vi "NI VeriStand FPGA Interface Tools Installer.vi"() -> ()   [LabVIEW 2010]
panel:
  out "Install Status":string
  in  "Uninstall":bool
  in  "Accept":bool
  out "License":string="Copyright (c) 2011, National Instruments\nAll rights reserved.\n\nRedistribution and use in source and binary forms, with or without modification, are permitted provided that the following conditions are met:\n\no Redistributions of source code must retain the above copyright notice, this list of conditions and the following disclaimer.\no Redistributions in binary form must reproduce the above copyright notice, this list of conditions and the following disclaimer in the documentation and/or other materials provided with the distribution.\no Neither the name of the National Instruments Corporation nor the names of its contributors may be used to endorse or promote products derived from this software without specific prior written permission.\n\nTHIS SOFTWARE IS PROVIDED BY THE COPYRIGHT HOLDERS AND CONTRIBUTORS \"AS IS\" AND ANY EXPRESS OR IMPLIED WARRANTIES, INCLUDING, BUT NOT LIMITED TO, THE IMPLIED WARRANTIES OF MERCHANTABILITY AND FITNESS FOR A PARTICULAR PURPOSE ARE DISCLAIMED. IN NO EVENT SHALL THE COPYRIGHT HOLDER OR CONTRIBUTORS BE LIABLE FOR ANY DIRECT, INDIRECT, INCIDENTAL, SPECIAL, EXEMPLARY, OR CONSEQUENTIAL DAMAGES (INCLUDING, BUT NOT LIMITED TO, PROCUREMENT OF SUBSTITUTE GOODS OR SERVICES; LOSS OF USE, DATA, OR PROFITS; OR BUSINESS INTERRUPTION) HOWEVER CAUSED AND ON ANY THEORY OF LIABILITY, WHETHER IN CONTRACT, STRICT LIABILITY, OR TORT (INCLUDING NEGLIGENCE OR OTHERWISE) ARISING IN ANY WAY OUT OF THE USE OF THIS SOFTWARE, EVEN IF ADVISED OF THE POSSIBILITY OF SUCH DAMAGE."
  in  "Cancel":bool
  in  "Install":bool
  # "NI VeriStand FPGA-Based I/O Interface Tools"
  # "1. Installs NI VeriStand FPGA project wizard to Getting Started Windows and New dialog.\n2. Installs NI VeriStand RIO Library, NI VeriStand FPGA Templates, palettes, and examples."
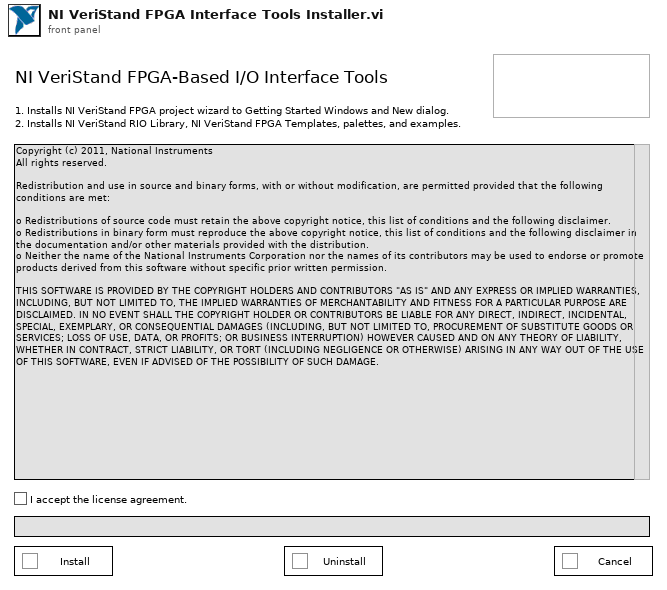
[diagram p1: front panel]
types:
  T1 = enum8{"Enabled", "Disabled", "Disabled and Grayed Out"}
  T2 = enum16{"copy files", "Xplatform copy", "move external linked files to temp", "mass compile", "move temp files to user.lib", "del mass comp proj"}
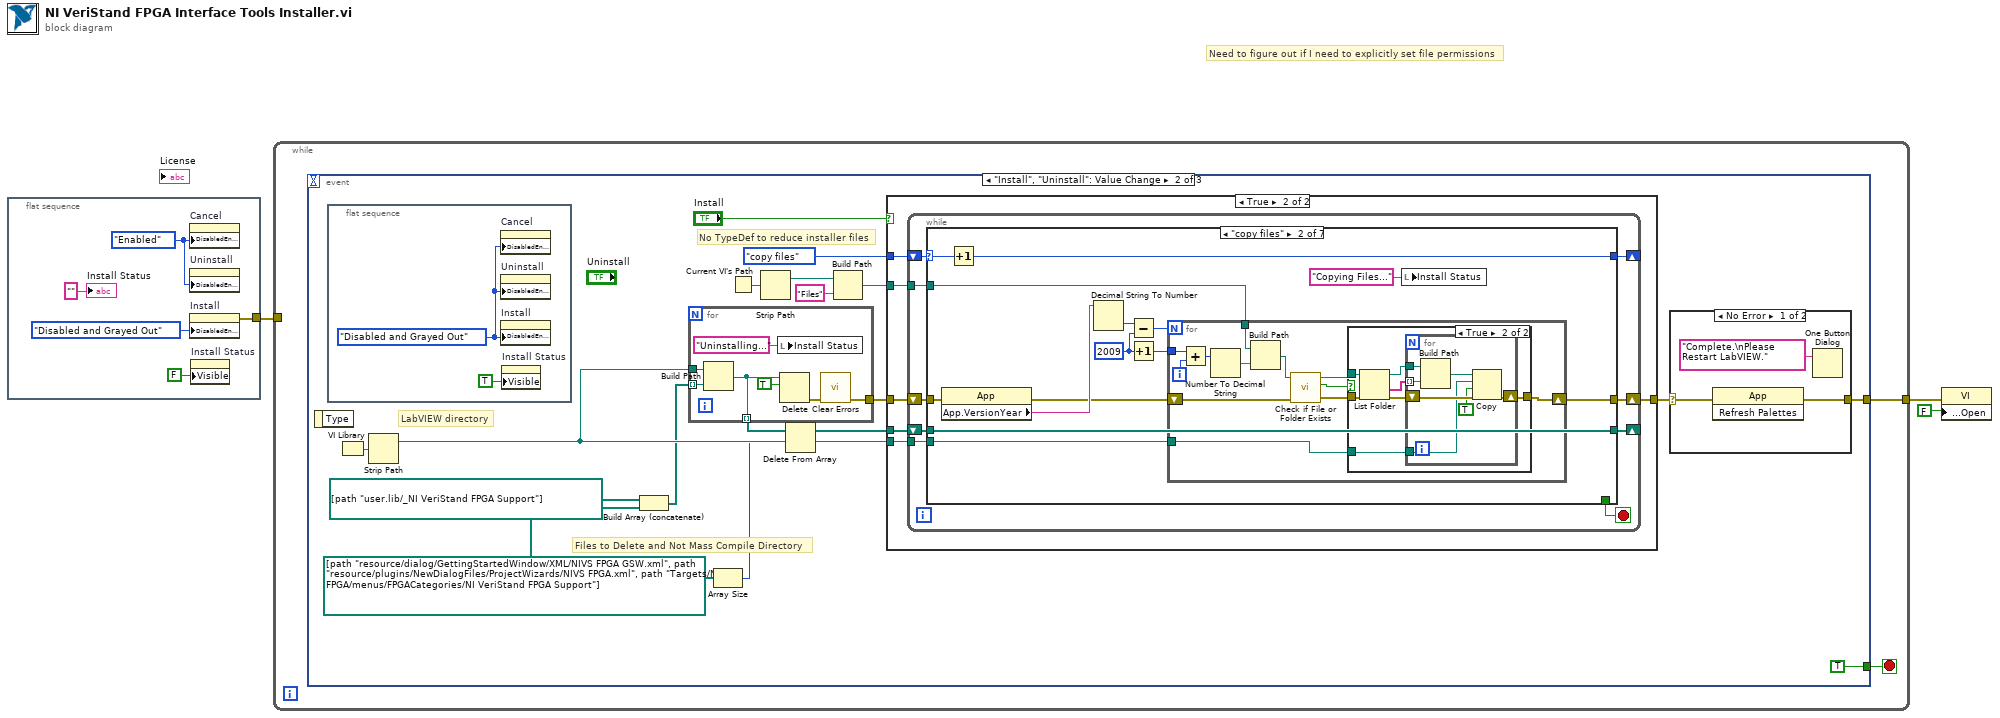
[diagram p0: block diagram]
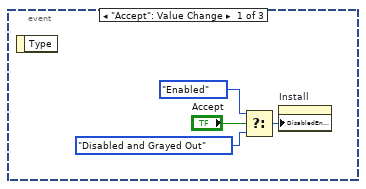
[diagram p2: hidden frame]
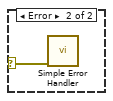
[diagram p3: hidden frame]
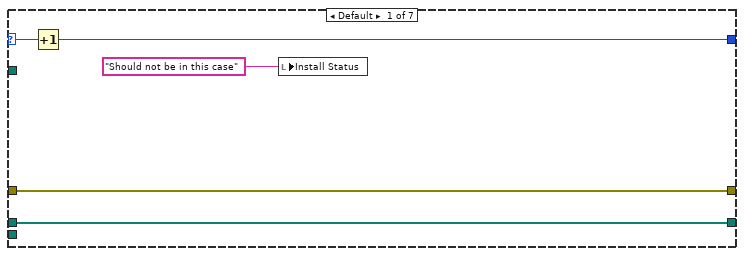
[diagram p5: hidden frame]
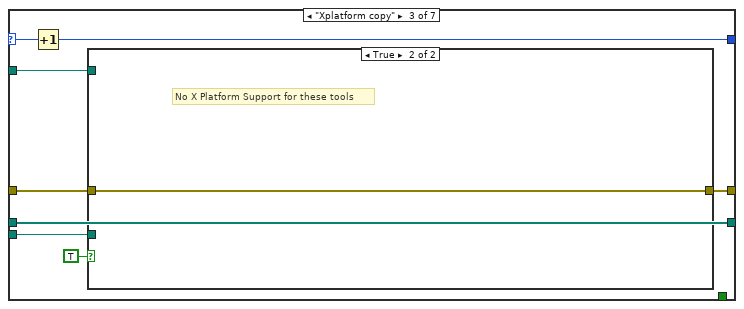
[diagram p7: hidden frame]
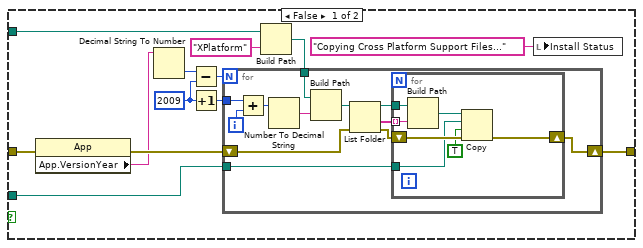
[diagram p8: hidden frame]
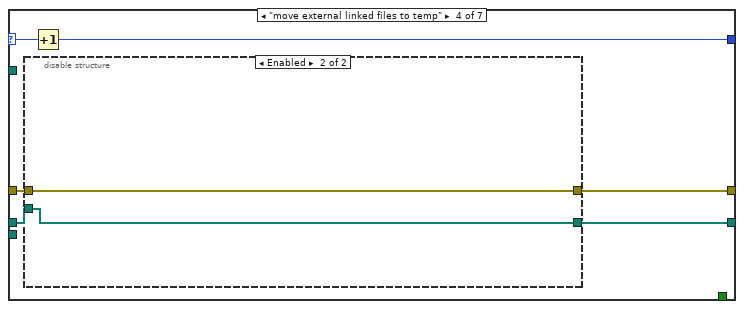
[diagram p9: hidden frame]
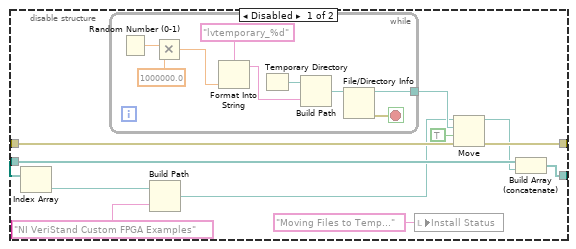
[diagram p10: hidden frame]
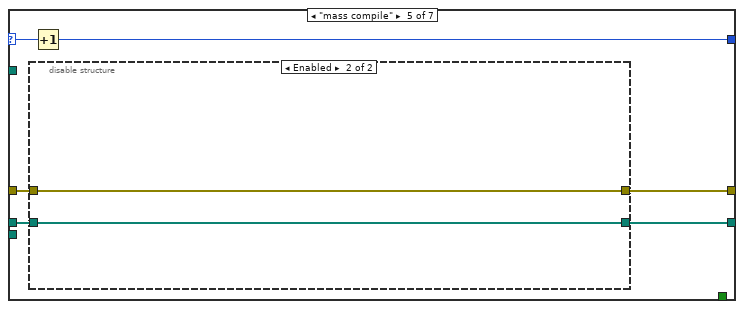
[diagram p11: hidden frame]
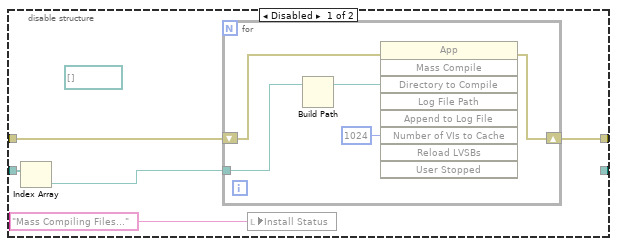
[diagram p12: hidden frame]
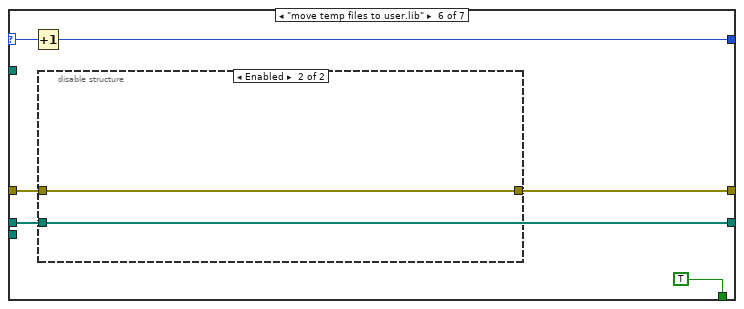
[diagram p13: hidden frame]
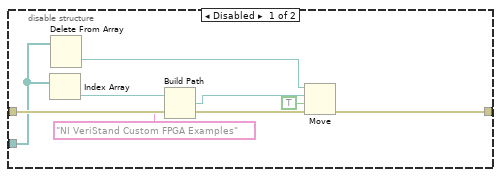
[diagram p14: hidden frame]
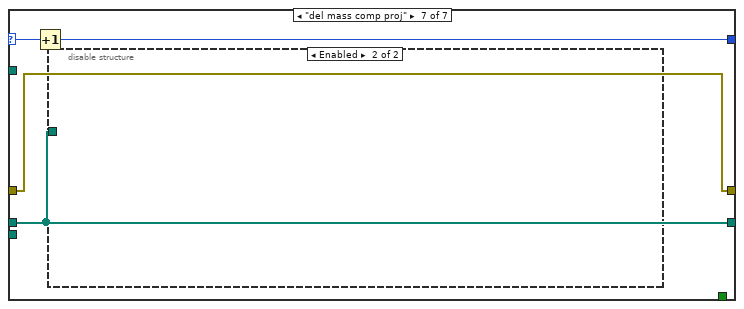
[diagram p15: hidden frame]
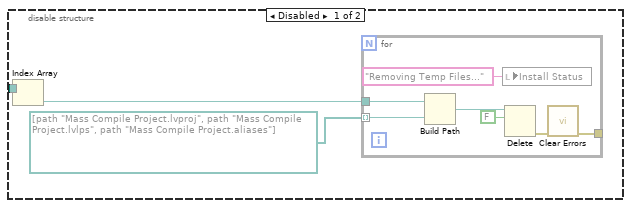
[diagram p16: hidden frame]
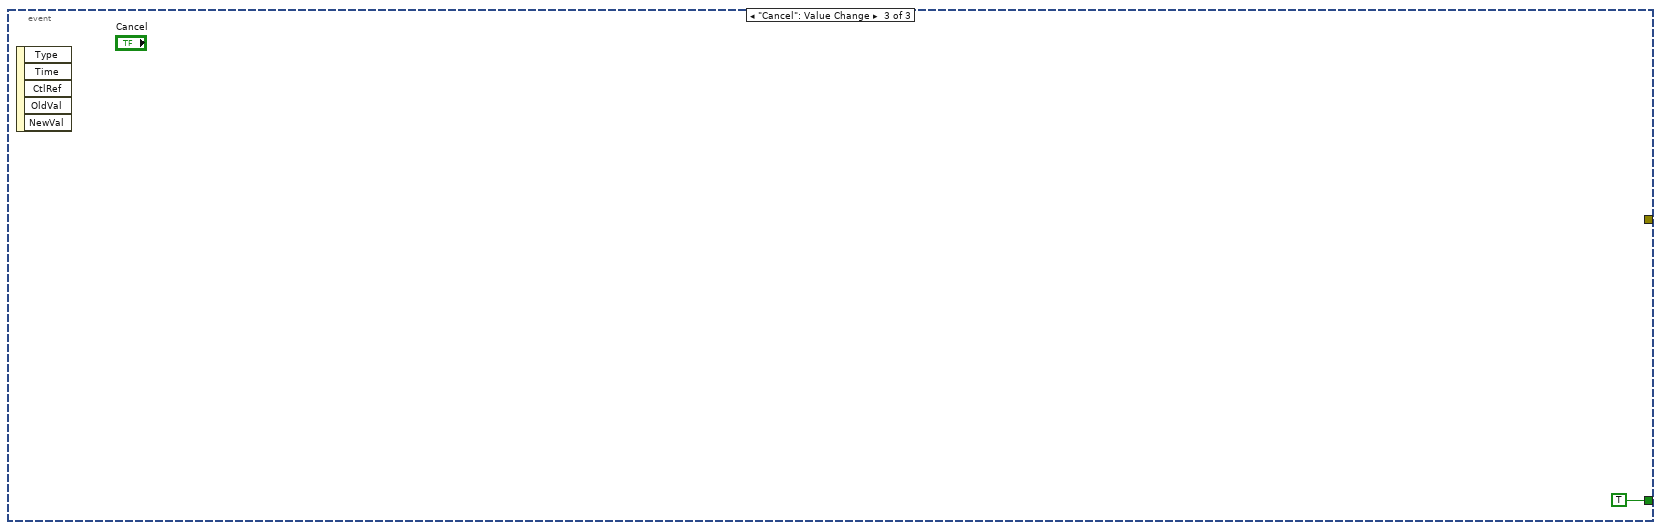
[diagram p17: hidden frame]
diagram:
  # "Need to figure out if I need to explicitly set file permissions"
  n1 = flat-sequence {
    tunnel: [w4] -> w3
    frame #0 {
      w8 = T1."Enabled" ("Disabled")
      n2 = property on="Cancel" class="Bool"("DisabledEnum"=w8) -> ()  [unwired: 2 in, 2 out]
      n3 = property on="Uninstall" class="Bool"("DisabledEnum"=w8) -> ()  [unwired: 2 in, 2 out]
      n4 = property on="Install" class="Bool"("DisabledEnum"=T1."Disabled and Grayed Out" ("Disabled")) -> (error out=w4:errorcluster)  [unwired: 2 in, 1 out]
      n5 = property on="Install Status" class="Str"("Visible"=FALSE) -> ()  [unwired: 2 in, 2 out]
      "Install Status" <- "" ("Install Status")
    }
  }
  n6 = while {
    tunnel: w3 -> [_]
    tunnel: [w9] -> w1
    stop <- w10 stop-if-true
    n7 = event shown="[1] \"Install\", \"Uninstall\": Value Change" {
      selector: _ -> [_ _ _]
      dyn-events: _ -> [_ _ _]
      timeout: _ -> [_ _ _]
      tunnel: [_ TRUE TRUE] -> w10
      tunnel: [_ w21 _] -> w9
      event "Accept": Value Change {
        n8 = event-data() -> ()  [unwired: 1 in, 1 out]
        n9 = Select(t=T1."Enabled" ("Disabled"), s="Accept", f=T1."Disabled and Grayed Out" ("Disabled")) -> (s? t:f=w12:T1)
        n10 = property on="Install" class="Bool"("DisabledEnum"=w12) -> ()  [unwired: 2 in, 2 out]
      }
      event "Install", "Uninstall": Value Change {
        w17 = path[] [path "resource/dialog/GettingStartedWindow/XML/NIVS FPGA GSW.xml", path "resource/plugins/NewDialogFiles/ProjectWizards/NIVS FPGA.xml", path "Targets/NI/FPGA/menus/FPGACategories/NI VeriStand FPGA Support"] ("element")
        # "Files to Delete and Not Mass Compile Directory"
        # "No TypeDef to reduce installer files"
        # "LabVIEW directory"
        n11 = event-data() -> ()  [unwired: 1 in, 1 out]
        n12 = flat-sequence {
          frame #0 {
            w223 = T1."Disabled and Grayed Out" ("Disabled")
            n13 = property on="Cancel" class="Bool"("DisabledEnum"=w223) -> ()  [unwired: 2 in, 2 out]
            n14 = property on="Uninstall" class="Bool"("DisabledEnum"=w223) -> ()  [unwired: 2 in, 2 out]
            n15 = property on="Install" class="Bool"("DisabledEnum"=w223) -> ()  [unwired: 2 in, 2 out]
            n16 = property on="Install Status" class="Str"("Visible"=TRUE) -> ()  [unwired: 2 in, 2 out]
          }
        }
        n17 = VI Library() -> (path=w31:path)
        n18 = Strip Path(path=w31) -> (stripped path=w23:path)  [unwired: 1 out]
        n19 = Build Array (concatenate)(path[] [path "user.lib/_NI VeriStand FPGA Support"], w17) -> (w19:path[])
        n20 = for {
          tunnel: w23 -> [w221]
          tunnel: w19 -> [w220] mode=indexing
          tunnel: [w216] -> w24
          tunnel: [w215] -> w20 mode=indexing
          n21 = Build Path(base path=w221, name or relative path=w220) -> (appended path=w215:path)
          n22 = local write "Install Status"("Uninstalling..." ("Install Status")) -> ()
          n23 = Delete(path (use dialog)=w215, entire hierarchy (F)=TRUE) -> (error out=w217:errorcluster)  [unwired: 3 in, 2 out]
          n24 = call <vilib>:"Clear Errors.vi"("error in (no error)"=w217) -> ("error out"=w216:errorcluster)  [unwired: 6 in]
        }
        n25 = Array Size(array=w17) -> (size(s)=w16:i32)
        n26 = Current VI's Path() -> (path=w30:path)
        n27 = Strip Path(path=w30) -> (stripped path=w29:path)  [unwired: 1 out]
        n28 = Delete From Array(array=w20, length=w16) -> (array with subset deleted=w18:path[])  [unwired: 1 in, 1 out]
        n29 = Build Path(base path=w29, name or relative path="Files") -> (appended path=w25:path)
        n30 = case shown="True" "Install" {
          tunnel: T2."copy files" -> [_ w43]
          tunnel: w25 -> [_ w42]
          tunnel: w24 -> [w37 w41]
          tunnel: w23 -> [_ w40]
          tunnel: w18 -> [_ w39]
          tunnel: [w37 w38] -> w22
          frame False {
          }
          frame True {
            n31 = while {
              shift-right: [w51] -> _
              shift-left: w43 -> [w52]
              tunnel: w42 -> [w49]
              shift-right: [w46] -> w38
              shift-left: w41 -> [w48]
              tunnel: w40 -> [w47]
              shift-right: [w44] -> _
              shift-left: w39 -> [w45]
              stop <- w50 stop-if-true
              n32 = case shown="\"copy files\"" w52 {
                selector: w52 -> [w57 w71 w106 w145 w173 w191 w204]
                tunnel: [w56 w70 w105 w144 w172 w190 w203] -> w51
                tunnel: [_ _ _ _ _ TRUE _] -> w50
                tunnel: w49 -> [_ w63 w104 _ _ _ _]
                tunnel: w48 -> [w53 w69 w101 w142 w171 w188 w201]
                tunnel: w47 -> [_ w62 w103 _ _ _ _]
                tunnel: [w53 w60 w102 w141 w170 w187 w201] -> w46
                tunnel: w45 -> [w54 w58 w100 w143 w169 w186 w202]
                tunnel: [w54 w58 w100 w140 w168 w186 w202] -> w44
                frame Default {
                  n33 = Increment(x=w57) -> (x+1=w56:T2)
                  n34 = local write "Install Status"("Should not be in this case" ("Install Status")) -> ()
                }
                frame "copy files" {
                  w65 = 2009 ("y")
                  n35 = property class="App"(error in=w69) -> (error out=w61:errorcluster, "App.VersionYear"=w68:string)  [unwired: 1 in, 1 out]
                  n36 = Increment(x=w71) -> (x+1=w70:T2)
                  n37 = Decimal String To Number(string=w68) -> (number=w67:i32)  [unwired: 2 in, 1 out]
                  n38 = Subtract(x=w67, y=w65) -> (x-y=w66:i32)
                  n39 = Increment(x=w65) -> (x+1=w64:i32)
                  n40 = for {
                    N: w66 -> [_]
                    tunnel: w64 -> [w83]
                    tunnel: w63 -> [w79]
                    tunnel: w62 -> [w78]
                    shift-right: [w76] -> w60
                    shift-left: w61 -> [w77]
                    i -> [w82]
                    n41 = Add(x=w83, y=w82) -> (x+y=w81:i32)
                    n42 = Number To Decimal String(number=w81) -> (decimal integer string=w80:string)  [unwired: 1 in]
                    n43 = Build Path(base path=w79, name or relative path=w80) -> (appended path=w74:path)
                    n44 = call <vilib>:"Check if File or Folder Exists.vi"("error in (no error)"=w77, "path"=w74) -> ("error out"=w75:errorcluster, "file or folder exists?"=w72:bool, "dup path"=w73:path)  [unwired: 7 in]
                    n45 = case shown="True" w72 {
                      tunnel: w73 -> [_ w88]
                      tunnel: w78 -> [_ w87]
                      tunnel: w75 -> [w84 w86]
                      tunnel: [w84 w85] -> w76
                      frame False {
                      }
                      frame True {
                        n46 = List Folder(path=w88, error in=w86) -> (path out=w90:path, folder names=w89:string[], error out=w91:errorcluster)  [unwired: 2 in, 1 out]
                        n47 = for {
                          tunnel: w89 -> [w97] mode=indexing
                          tunnel: w90 -> [w98]
                          shift-right: [w92] -> w85
                          shift-left: w91 -> [w95]
                          tunnel: w87 -> [w93]
                          n48 = Build Path(base path=w98, name or relative path=w97) -> (appended path=w96:path)
                          n49 = Copy(8:w95, 9:TRUE ("overwrite (F)"), 10:w93, 11:w96) -> (0:w92:errorcluster)  [unwired: 1 in, 2 out]
                        }
                      }
                    }
                  }
                  n50 = local write "Install Status"("Copying Files..." ("Install Status")) -> ()
                }
                frame "Xplatform copy" {
                  n51 = Increment(x=w106) -> (x+1=w105:T2)
                  n52 = case shown="True" TRUE {
                    tunnel: w104 -> [w112 _]
                    tunnel: w103 -> [w115 _]
                    tunnel: w101 -> [w109 w139]
                    tunnel: [w114 w139] -> w102
                    frame False {
                      w117 = 2009 ("y")
                      n53 = property class="App"(error in=w109) -> (error out=w108:errorcluster, "App.VersionYear"=w107:string)  [unwired: 1 in, 1 out]
                      n54 = Decimal String To Number(string=w107) -> (number=w119:i32)  [unwired: 2 in, 1 out]
                      n55 = Subtract(x=w119, y=w117) -> (x-y=w118:i32)
                      n56 = Increment(x=w117) -> (x+1=w116:i32)
                      n57 = Build Path(base path=w112, name or relative path="XPlatform") -> (appended path=w111:path)
                      n58 = for {
                        N: w118 -> [_]
                        tunnel: w116 -> [w131]
                        tunnel: w111 -> [w127]
                        tunnel: w115 -> [w122]
                        shift-right: [w120] -> w114
                        shift-left: w108 -> [w121]
                        i -> [w130]
                        n59 = Add(x=w131, y=w130) -> (x+y=w129:i32)
                        n60 = Number To Decimal String(number=w129) -> (decimal integer string=w128:string)  [unwired: 1 in]
                        n61 = Build Path(base path=w127, name or relative path=w128) -> (appended path=w123:path)
                        n62 = List Folder(path=w123, error in=w121) -> (path out=w125:path, folder names=w124:string[], error out=w126:errorcluster)  [unwired: 2 in, 1 out]
                        n63 = for {
                          tunnel: w124 -> [w137] mode=indexing
                          tunnel: w125 -> [w138]
                          shift-right: [w132] -> w120
                          shift-left: w126 -> [w135]
                          tunnel: w122 -> [w133]
                          n64 = Build Path(base path=w138, name or relative path=w137) -> (appended path=w136:path)
                          n65 = Copy(8:w135, 9:TRUE ("overwrite (F)"), 10:w133, 11:w136) -> (0:w132:errorcluster)  [unwired: 1 in, 2 out]
                        }
                      }
                      n66 = local write "Install Status"("Copying Cross Platform Support Files..." ("Install Status")) -> ()
                    }
                    frame True {
                      # "No X Platform Support for these tools"
                    }
                  }
                }
                frame "move external linked files to temp" {
                  n67 = disable-structure shown="Enabled" {
                    disable-tunnel: w143 -> [w156 w167]
                    disable-tunnel: w142 -> [w155 w166]
                    disable-tunnel: [w154 w166] -> w141
                    disable-tunnel: [w153 w167] -> w140
                    frame Disabled {
                      n68 = Index Array(array=w156) -> (element=w152:path)  [unwired: 1 in]
                      n69 = while {
                        tunnel: [w157] -> w150
                        stop <- w158 stop-if-true
                        n70 = Random Number (0-1)() -> (number: 0 to 1=w165:dbl)
                        n71 = Multiply(x=w165, y=1000000.0) -> (x*y=w162:dbl)
                        n72 = Format Into String(format string="lvtemporary_%d", w162) -> (resulting string=w161:string)  [unwired: 2 in, 1 out]
                        n73 = Temporary Directory() -> (w160:path)
                        n74 = Build Path(base path=w160, name or relative path=w161) -> (appended path=w159:path)
                        n75 = File/Directory Info(path=w159) -> (path out=w157:path, error out=w158:errorcluster)  [unwired: 1 in, 5 out]
                      }
                      n76 = Build Path(base path=w152, name or relative path="NI VeriStand Custom FPGA Examples") -> (appended path=w149:path)
                      n77 = local write "Install Status"("Moving Files to Temp..." ("Install Status")) -> ()
                      n78 = Move(source path=w149, error in=w155, 9:TRUE ("overwrite (F)"), 10:w150) -> (error out=w154:errorcluster, 3:w147:path)  [unwired: 1 in, 1 out]
                      n79 = Build Array (concatenate)(w156, w147) -> (w153:path[])
                    }
                    frame Enabled {
                    }
                  }
                  n80 = Increment(x=w145) -> (x+1=w144:T2)
                }
                frame "mass compile" {
                  n81 = disable-structure shown="Enabled" {
                    disable-tunnel: w171 -> [w177 w184]
                    disable-tunnel: [w176 w184] -> w170
                    disable-tunnel: w169 -> [w175 w185]
                    disable-tunnel: [_ w185] -> w168
                    frame Disabled {
                      (unwired) path[] []
                      n82 = Index Array(array=w175) -> (element=w174:path)  [unwired: 1 in]
                      n83 = for {
                        shift-right: [w182] -> w176
                        shift-left: w177 -> [w183]
                        tunnel: w174 -> [w179]
                        n84 = Build Path(base path=w179) -> (appended path=w180:path)  [unwired: 1 in]
                        n85 = invoke class="App" method="Mass Compile"(error in=w183, "Directory to Compile"=w180, "Number of VIs to Cache"=u32 1024) -> (error out=w182:errorcluster)  [unwired: 6 in, 8 out]
                      }
                      n86 = local write "Install Status"("Mass Compiling Files..." ("Install Status")) -> ()
                    }
                    frame Enabled {
                    }
                  }
                  n87 = Increment(x=w173) -> (x+1=w172:T2)
                }
                frame "move temp files to user.lib" {
                  n88 = Increment(x=w191) -> (x+1=w190:T2)
                  n89 = disable-structure shown="Enabled" {
                    disable-tunnel: w188 -> [w199 w200]
                    disable-tunnel: [w198 w200] -> w187
                    disable-tunnel: w186 -> [w197 _]
                    frame Disabled {
                      n90 = Index Array(array=w197) -> (element=w194:path)  [unwired: 1 in]
                      n91 = Delete From Array(array=w197) -> (deleted portion=w193:path)  [unwired: 2 in, 1 out]
                      n92 = Build Path(base path=w194, name or relative path="NI VeriStand Custom FPGA Examples") -> (appended path=w195:path)
                      n93 = Move(source path=w193, error in=w199, 9:TRUE ("overwrite (F)"), 10:w195) -> (error out=w198:errorcluster)  [unwired: 1 in, 2 out]
                    }
                    frame Enabled {
                    }
                  }
                }
                frame "del mass comp proj" {
                  n94 = Increment(x=w204) -> (x+1=w203:T2)
                  n95 = disable-structure shown="Enabled" {
                    disable-tunnel: w202 -> [w207 _]
                    frame Disabled {
                      n96 = Index Array(array=w207) -> (element=w206:path)  [unwired: 1 in]
                      n97 = for {
                        tunnel: w206 -> [w214]
                        tunnel: path[] [path "Mass Compile Project.lvproj", path "Mass Compile Project.lvlps", path "Mass Compile Project.aliases"] -> [w213] mode=indexing
                        tunnel: [w209] -> _
                        n98 = Build Path(base path=w214, name or relative path=w213) -> (appended path=w208:path)
                        n99 = local write "Install Status"("Removing Temp Files..." ("Install Status")) -> ()
                        n100 = Delete(path (use dialog)=w208, entire hierarchy (F)=FALSE) -> (error out=w210:errorcluster)  [unwired: 3 in, 2 out]
                        n101 = call <vilib>:"Clear Errors.vi"("error in (no error)"=w210) -> ("error out"=w209:errorcluster)  [unwired: 6 in]
                      }
                    }
                    frame Enabled {
                    }
                  }
                }
              }
            }
          }
        }
        n102 = case shown="No Error" w22 {
          selector: w22 -> [w34 w36]
          tunnel: [w33 _] -> w21
          frame No Error {
            n103 = invoke class="App" method="Refresh Palettes"(error in=w34) -> (error out=w33:errorcluster)  [unwired: 2 in, 2 out]
            n104 = One Button Dialog(message="Complete.\nPlease Restart LabVIEW." ("Install Status")) -> ()  [unwired: 1 in, 1 out]
          }
          frame Error {
            n105 = call <vilib>:"Simple Error Handler.vi"("error in (no error)"=w36) -> ()  [unwired: 4 in, 5 out]
          }
        }
      }
      event "Cancel": Value Change {
        n106 = event-data() -> ()  [unwired: 1 in, 5 out]
      }
    }
  }
  n107 = property class="VI"(error in=w1, "Front Panel.Open"=FALSE ("Front Panel Window:Open")) -> ()  [unwired: 1 in, 2 out]
